vi "Init List Panels.vi"(8 "error in (no error)":errorcluster, 11 "picoG in":refnum<class "picoG.lvclass">) -> (0 "error out":errorcluster, 3 "picoG out":refnum<class "picoG.lvclass">)   [LabVIEW 2020, in "PicoG-App.lvlib" / "picoG.lvclass"]
uses:
  picoG.lvclass
  AppListPanel/AppListPanel.lvclass
  C:/Program Files (x86)/National Instruments/LabVIEW 2020/vi.lib/IlluminatedG/IG OOPanel/OOPanel/Panel/Panel.lvclass
  DeviceListPanel/DeviceListPanel.lvclass
  PlatformListPanel/PlatformListPanel.lvclass
  picoG.lvclass/picoG.ctl
  <vilib>/IlluminatedG/IG OOPanel/OOPanel/Manager/Manager.lvclass
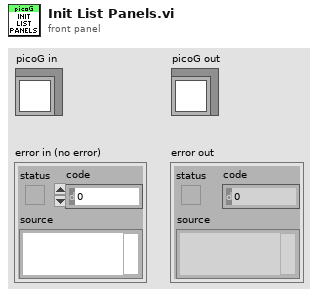
[diagram p1: front panel]
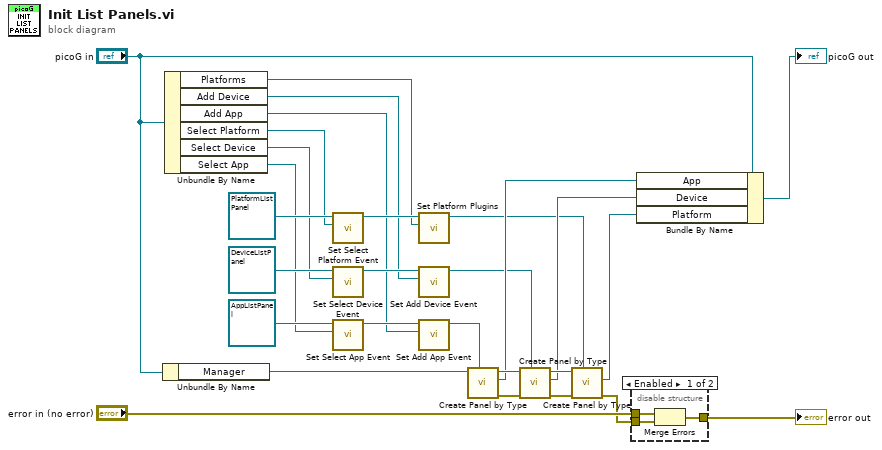
[diagram p0: block diagram]
diagram:
  n1 = Unbundle By Name("picoG in") -> ("Manager"=w17:refnum<class "Manager.lvclass">)
  n2 = Unbundle By Name("picoG in") -> ("Platforms"=w7:refnum<class "PlatformManager.lvclass">, "Add Device"=w9:refnum<user-event>, "Add App"=w1:refnum<user-event>, "Select Platform"=w5:refnum<user-event>, "Select Device"=w6:refnum<user-event>, "Select App"=w4:refnum<user-event>)
  n3 = call "Set Select Platform Event.vi"("Select Platform"=w5, "PlatformListPanel in"=refnum<class "PlatformListPanel.lvclass"> refnum ("PicoG-App.lvlib:PlatformListPanel.lvclass")) -> ("PlatformListPanel out"=w12:refnum<class "PlatformListPanel.lvclass">)  [unwired: 8 in, 1 out]
  n4 = call "Set Select Device Event.vi"("Select Device"=w6, "DeviceListPanel in"=refnum<class "DeviceListPanel.lvclass"> refnum ("PicoG-App.lvlib:DeviceListPanel.lvclass")) -> ("DeviceListPanel out"=w10:refnum<class "DeviceListPanel.lvclass">)  [unwired: 8 in, 1 out]
  n5 = call "Set Select App Event.vi"("Select App"=w4, "AppListPanel in"=refnum<class "AppListPanel.lvclass"> refnum ("PicoG-App.lvlib:AppListPanel.lvclass")) -> ("AppListPanel out"=w3:refnum<class "AppListPanel.lvclass">)  [unwired: 8 in, 1 out]
  n6 = call "Set Platform Plugins.vi"("Platform Plugins"=w7, "PlatformListPanel in"=w12) -> ("PlatformListPanel out"=w21:refnum<class "PlatformListPanel.lvclass">)  [unwired: 8 in, 1 out]
  n7 = call "Set Add Device Event.vi"("Add Device"=w9, "DeviceListPanel in"=w10) -> ("DeviceListPanel out"=w8:refnum<class "DeviceListPanel.lvclass">)  [unwired: 8 in, 1 out]
  n8 = call "Set Add App Event.vi"("Add App"=w1, "AppListPanel in"=w3) -> ("AppListPanel out"=w2:refnum<class "AppListPanel.lvclass">)  [unwired: 8 in, 1 out]
  n9 = call <vilib>:"Create Panel by Type.vi"("Panel Type"=w2, "Manager in"=w17) -> ("error out"=w16:errorcluster, "Panel"=w22:refnum<class "AppListPanel.lvclass">, "Manager out"=w27:refnum<class "Manager.lvclass">)  [unwired: 7 in]
  n10 = call <vilib>:"Create Panel by Type.vi"("Panel Type"=w8, "error in (no error)"=w16, "Manager in"=w27) -> ("error out"=w15:errorcluster, "Panel"=w23:refnum<class "DeviceListPanel.lvclass">, "Manager out"=w26:refnum<class "Manager.lvclass">)  [unwired: 6 in]
  n11 = call <vilib>:"Create Panel by Type.vi"("Panel Type"=w21, "error in (no error)"=w15, "Manager in"=w26) -> ("error out"=w13:errorcluster, "Panel"=w24:refnum<class "PlatformListPanel.lvclass">)  [unwired: 6 in, 1 out]
  n12 = disable-structure shown="Enabled" {
    disable-tunnel: "error in (no error)" -> [w31 w32]
    disable-tunnel: [w30 w32] -> w14
    disable-tunnel: w13 -> [w29 _]
    frame Enabled {
      n13 = Merge Errors(w31, w29) -> (w30:errorcluster)
    }
    frame Disabled {
    }
  }
  "error out" <- w14
  n14 = Bundle By Name(cluster="picoG in", "App"=w22, "Device"=w23, "Platform"=w24) -> (→"picoG out":refnum<class "picoG.lvclass">)
